vi "Measure all.vi"(8 "error in (no error)":errorcluster, 11 "Power Supplies in":refnum<class "Power Supply.lvclass">[](array[class])) -> (0 "error out":errorcluster, 2 "Measurements":T1[](array[typedef]), 3 "Power Supplies out":refnum<class "Power Supply.lvclass">[](array[class]), 4 "Currents (A)":dbl[](array[numeric]), 6 "Voltages (V)":dbl[](array[numeric]))   [LabVIEW 2020, in "Power Supply.lvclass"]
uses:
  Power Supply.lvclass
  XML Handler/Controls/Result Cluster.ctl
  XML Handler/XML Handler.lvclass
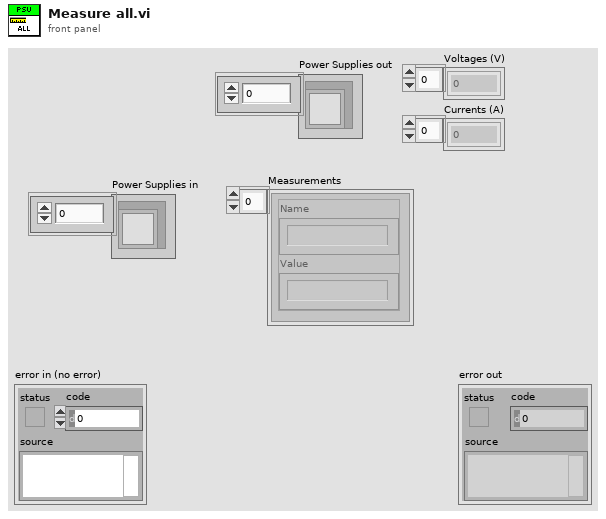
[diagram p1: front panel]
types:
  T1 = typedef "XML Handler.lvclass/Result Cluster.ctl" = cluster{"Name":string, "Value":string}
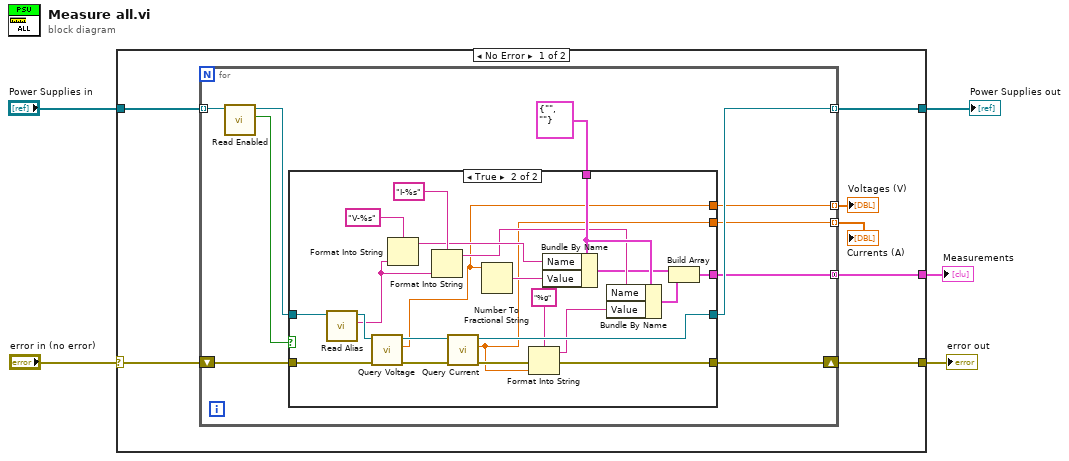
[diagram p0: block diagram]
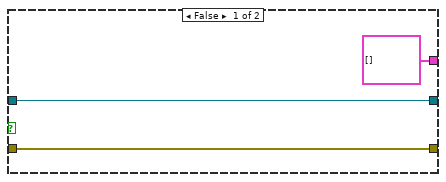
[diagram p2: hidden frame]
diagram:
  n1 = case shown="No Error" "error in (no error)" {
    selector: "error in (no error)" -> [w12 w49]
    tunnel: [w11 w49] -> w4
    tunnel: [w9 w48] -> w2
    tunnel: "Power Supplies in" -> [w10 w48]
    tunnel: [w8 _] -> w1
    frame No Error {
      n2 = for {
        tunnel: w10 -> [w18] mode=indexing
        tunnel: [w17] -> w9 mode=indexing
        shift-right: [w21] -> w11
        shift-left: w12 -> [w22]
        tunnel: [w15] -> w8 mode=concatenating
        tunnel: [w14] -> w7 mode=indexing
        tunnel: [w13] -> w6 mode=indexing
        n3 = call-dynamic "Read Enabled.vi"("Power Supply in"=w18) -> ("Enabled"=w20:bool, "Power Supply out"=w19:refnum<class "Power Supply.lvclass">)  [unwired: 9 in]
        n4 = case shown="True" w20 {
          tunnel: [w24 w46] -> w17
          tunnel: w22 -> [w23 w43]
          tunnel: T1 {"Name"="", "Value"=""} ("Result Cluster") -> [_ w37]
          tunnel: [w23 w28] -> w21
          tunnel: [T1[] [] w33] -> w15
          tunnel: w19 -> [w24 w32]
          tunnel: [_ w27] -> w13
          tunnel: [_ w26] -> w14
          frame False {
          }
          frame True {
            n5 = call-dynamic "Read Alias.vi"("Power Supply in"=w32) -> ("Alias"=w40:string, "Power Supply out"=w44:refnum<class "Power Supply.lvclass">)  [unwired: 9 in]
            n6 = call-dynamic "Query Voltage.vi"("error in (no error)"=w43, "Power Supply in"=w44) -> ("error out"=w45:errorcluster, "Voltage"=w26:dbl, "Power Supply out"=w47:refnum<class "Power Supply.lvclass">)  [unwired: 7 in]
            n7 = Format Into String(format string="V-%s", w40) -> (resulting string=w39:string)  [unwired: 2 in, 1 out]
            n8 = Format Into String(format string="I-%s", w40) -> (resulting string=w36:string)  [unwired: 2 in, 1 out]
            n9 = call-dynamic "Query Current.vi"("error in (no error)"=w45, "Power Supply in"=w47) -> ("error out"=w29:errorcluster, "Current"=w27:dbl, "Power Supply out"=w46:refnum<class "Power Supply.lvclass">)  [unwired: 7 in]
            n10 = Number To Fractional String(number=w26) -> (F-format string=w38:string)  [unwired: 3 in]
            n11 = Format Into String(format string="%g", error in=w29, w27) -> (resulting string=w30:string, error out=w28:errorcluster)  [unwired: 1 in]
            n12 = Bundle By Name(cluster=w37, "Name"=w39, "Value"=w38) -> (w35:T1)
            n13 = Bundle By Name(cluster=w37, "Name"=w36, "Value"=w30) -> (w34:T1)
            n14 = Build Array(w35, w34) -> (w33:T1[])
          }
        }
      }
      "Voltages (V)" <- w7
      "Currents (A)" <- w6
    }
    frame Error {
    }
  }
  "error out" <- w4
  "Power Supplies out" <- w2
  "Measurements" <- w1
